vi "Set Y Tovey.vi"(10 "Y Tovey":refnum<class "Tovey 9150.lvclass">, 11 "Model in":refnum<class "Model.lvclass">) -> (3 "Model out":refnum<class "Model.lvclass">)   [LabVIEW 2016]
uses:
  Model.lvclass
  TEI-9150/Tovey 9150.lvclass
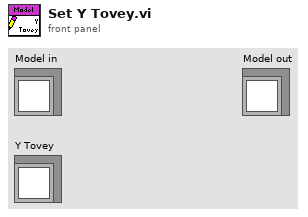
[diagram p1: front panel]
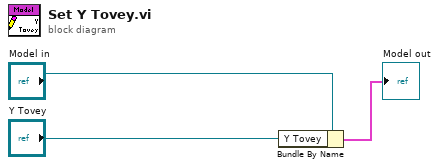
[diagram p0: block diagram]
diagram:
  n1 = Bundle By Name(cluster="Model in", "Y Tovey"="Y Tovey") -> (→"Model out":cluster{})
